vi "UDP Data Link - Driver Utilities - Asynch UDP Loop.vi"(11 "Input Data":T1) -> ()   [LabVIEW 2012, in "UDP Data Link Engine.lvlib"]
doc: "This VI is launched dynamically in its own memory space from the inline model VI. Before running, the Input Data control is initialized with UDP information entered by the user in System Explorer and with the appropriate RT FIFOs and Status Notifier.\n\nThis VI waits for data from an RT FIFO, converts the data to the appropriate packet data, and writes the packet over UDP to a Simulation Machine. The Simulation Machine responds with a UDP packet of its own, which this VI is monitoring in a separate loop. Upon receving UDP packets, this VI converts it to the appropriate data, determines any errors, and writes this data to the inline model VI via RT FIFO."
uses:
  UDP Data Link Engine.lvlib
  <vilib>/NI Veristand/Custom Device Tools/Custom Device Utility Library/Custom Device Utility Library.lvlib
panel:
  in  "Protocol Info":cluster{"ProtocolId":u8, "ProtocolRev":u8}={"ProtocolId"=1, "ProtocolRev"=16} {"ProtocolRev" format="%b"; "ProtocolId" format="%b"}
  # "If protocol info is rev'd, modify this cluster and then save as defualut data."
  # "From RT Driver VI"
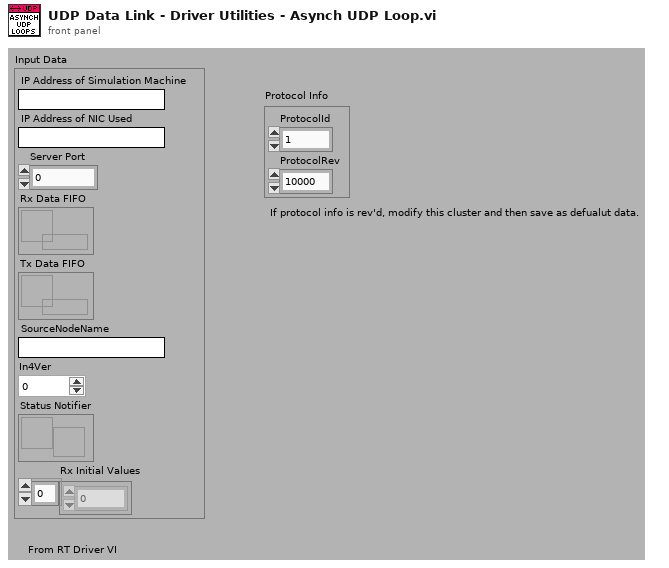
[diagram p1: front panel]
types:
  T1 = cluster{"IP Address of Simulation Machine":string, "IP Address of NIC Used":string, "Server Port":u16, "Rx Data FIFO":refnum<k33>, "Tx Data FIFO":refnum<k33>, "SourceNodeName":string, "In4Ver":u16, "Status Notifier":refnum<notifier>, "Rx Initial Values":dbl[]}
  T2 = enum16{"big-endian, network order", "native, host order", "little-endian"}
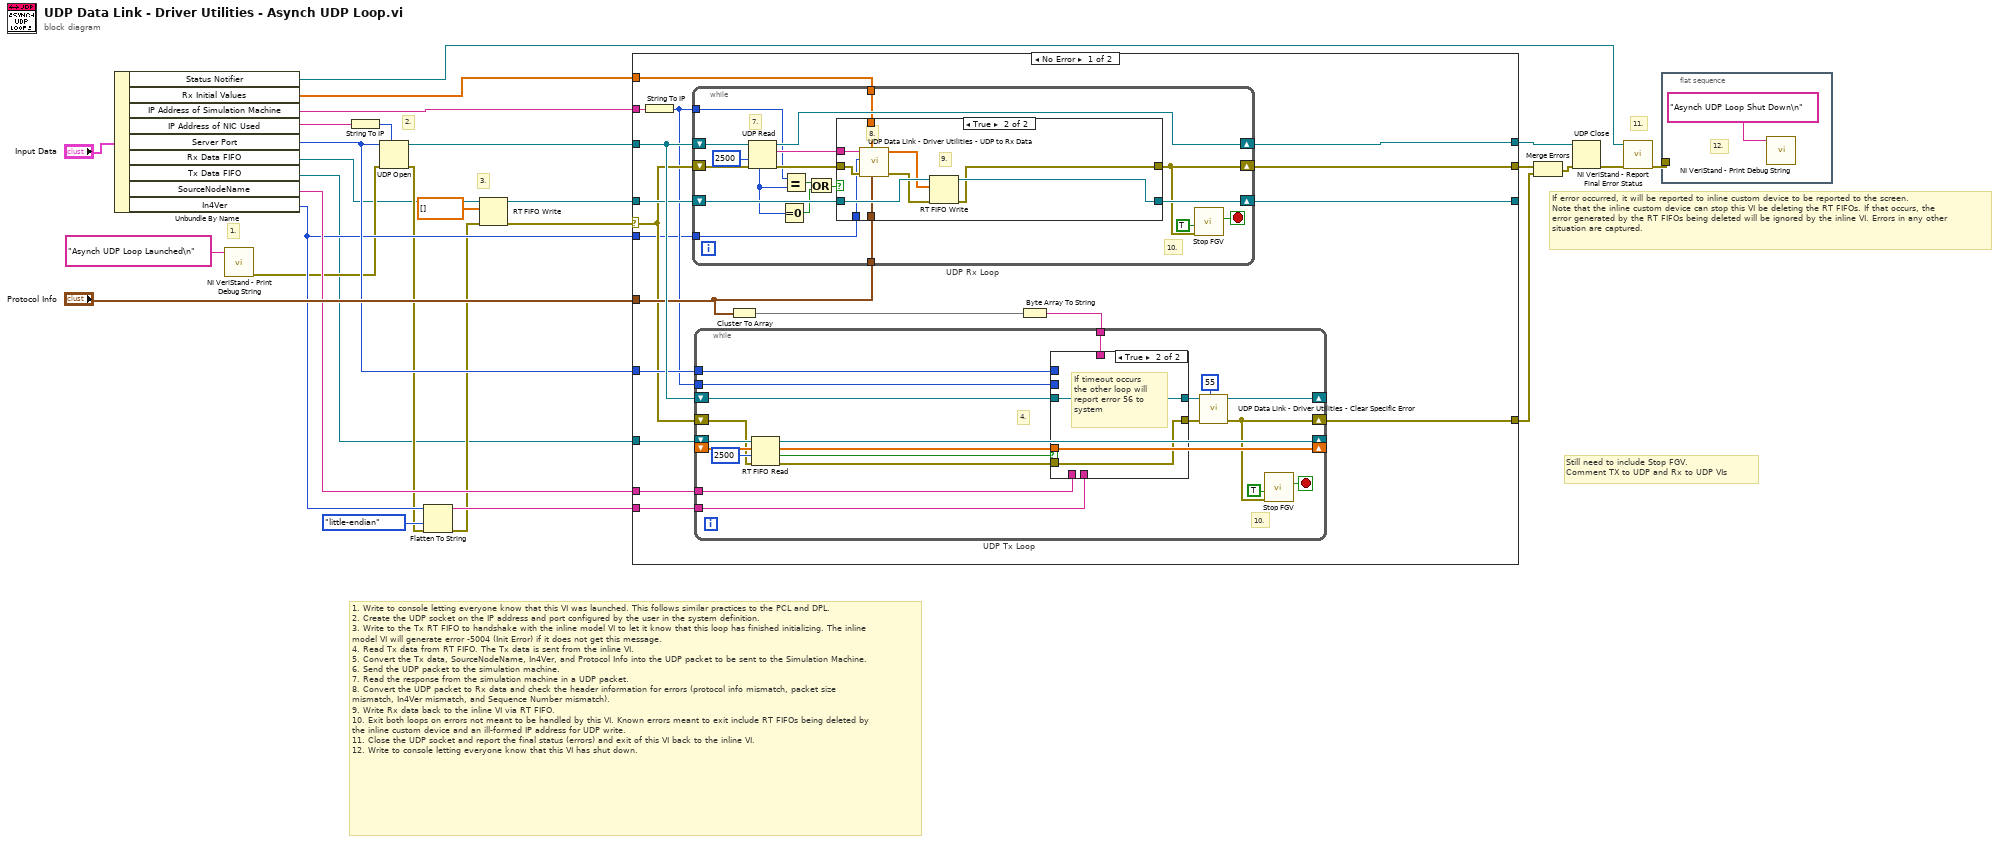
[diagram p0: block diagram]
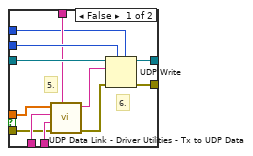
[diagram p2: hidden frame]
diagram:
  # "Still need to include Stop FGV.\nComment TX to UDP and Rx to UDP VIs"
  # "11."
  # "1. Write to console letting everyone know that this VI was launched. This follows similar practices to the PCL and DPL.\n2. Create the UDP socket on the IP address and port configured by the user in the system definition.\n3. Write to the Tx RT FIFO to handshake with the inline model VI to let it know that this loop has finished initializing. The inline model VI will generate error -5004 (Init Error) if it does not get this message.\n4. Read Tx data from RT FIFO. The Tx data is sent from the inline VI.\n5. Convert the Tx data, SourceNodeName, In4Ver, and Protocol Info into the UDP packet to be sent to the Simulation Machine.\n6. Send the UDP packet to the simulation machine.\n7. Read the response from the simulation machine in a UDP packet.\n8. Convert the UDP packet to Rx data and check the header information for errors (protocol info mismatch, packet size mismatch, In4Ver mismatch, and Sequence Number mismatch).\n9. Write Rx data back to the inline VI via RT FIFO.\n10. Exit both loops on errors not meant to be handled by this VI. Known errors meant to exit include RT FIFOs being deleted by the inline custom device and an ill-formed IP address for UDP write.\n11. Close the UDP socket and report the final status (errors) and exit of this VI back to the inline VI.\n12. Write to console letting everyone know that this VI has shut down."
  # "3."
  # "2."
  # "1."
  # "If error occurred, it will be reported to inline custom device to be reported to the screen.\nNote that the inline custom device can stop this VI be deleting the RT FIFOs. If that occurs, the error generated by the RT FIFOs being deleted will be ignored by the inline VI. Errors in any other situation are captured."
  n1 = Unbundle By Name("Input Data") -> ("Status Notifier"=w3:refnum<notifier>, "Rx Initial Values"=w2:dbl[], "IP Address of Simulation Machine"=w17:string, "IP Address of NIC Used"=w27:string, "Server Port"=w15:u16, "Rx Data FIFO"=w5:refnum<k33>, "Tx Data FIFO"=w4:refnum<k33>, "SourceNodeName"=w24:string, "In4Ver"=w14:u16)
  n2 = call <vilib>:"NI VeriStand - Print Debug String.vi"("Message"="Asynch UDP Loop Launched\n" ("String to write")) -> ("error out"=w8:errorcluster)  [unwired: 10 in]
  n3 = String To IP(1:w27) -> (0:w16:u32)
  n4 = UDP Open(7:w16, 8:w8, 11:w15) -> (port=w26:refnum<k16>, 0:w7:errorcluster)  [unwired: 2 in, 1 out]
  n5 = Flatten To String(anything=w14, byte order (0:big-endian, network order)=T2."little-endian", error in (no error)=w7) -> (data string=w23:string, error out=w6:errorcluster)  [unwired: 1 in, 1 out]
  n6 = RT FIFO Write(0:w5, 1:dbl[] [] ("element"), 3:w6) -> (8:w21:refnum<k33>, 11:w1:errorcluster)  [unwired: 2 in, 2 out]
  n7 = case shown="No Error" w1 {
    selector: w1 -> [w37 w113]
    tunnel: w26 -> [w46 w114]
    tunnel: w4 -> [w45 _]
    tunnel: w17 -> [w35 _]
    tunnel: "Protocol Info" -> [w44 _]
    tunnel: w24 -> [w41 _]
    tunnel: w23 -> [w40 _]
    tunnel: w15 -> [w39 _]
    tunnel: w21 -> [w38 w112]
    tunnel: [w36 w114] -> w18
    tunnel: w14 -> [w33 _]
    tunnel: [w32 w113] -> w13
    tunnel: [w31 w113] -> w12
    tunnel: [w30 w112] -> _
    tunnel: w2 -> [w29 _]
    frame No Error {
      n8 = String To IP(1:w35) -> (0:w34:u32)
      n9 = while "UDP Rx Loop" {
        shift-right: [w83] -> w32
        shift-left: w37 -> [w91]
        shift-right: [w93] -> w30
        shift-left: w38 -> [w98]
        shift-right: [w94] -> w36
        shift-left: w46 -> [w99]
        tunnel: w34 -> [w90]
        tunnel: w44 -> [w92]
        tunnel: w33 -> [w89]
        tunnel: w29 -> [w84]
        stop <- w82 stop-if-true
        # "10."
        # "7."
        n10 = UDP Read(connection ID=w99, timeout ms (25000)=2500, 8:w91) -> (data out=w95:string, error out=w96:errorcluster, 3:w94:refnum<k16>, 6:w85:u32)  [unwired: 1 in, 1 out]
        n11 = Equal To 0?(x=w85) -> (x = 0?=w86:bool)
        n12 = Equal?(x=w90, y=w85) -> (x = y?=w87:bool)
        n13 = Or(x=w87, y=w86) -> (x .or. y?=w88:bool)
        n14 = case shown="True" w88 {
          tunnel: w98 -> [w101 w111]
          tunnel: w96 -> [w100 w108]
          tunnel: w95 -> [_ w109]
          tunnel: [w101 w110] -> w93
          tunnel: [w100 w102] -> w83
          tunnel: w92 -> [_ w105]
          tunnel: w89 -> [_ w104]
          tunnel: w84 -> [_ w103]
          frame False {
          }
          frame True {
            # "9."
            # "8."
            n15 = call "UDP Data Link - Driver Utilities - UDP to Rx Data.vi"("Protocol Info"=w105, "Rx Initial Values"=w103, "error in (no error)"=w108, "In4Ver"=w104, "UDP Data"=w109) -> ("error out"=w106:errorcluster, "Rx Data"=w107:dbl[])  [unwired: 4 in, 1 out]
            n16 = RT FIFO Write(0:w111, 1:w107, 3:w106) -> (8:w110:refnum<k33>, 11:w102:errorcluster)  [unwired: 2 in, 2 out]
          }
        }
        n17 = call "Stop FGV.vi"("error in (no error)"=w83, "Stop on Error?"=TRUE) -> ("Latched Stop"=w82:bool)  [unwired: 7 in, 2 out]
      }
      n18 = Cluster To Array(cluster=w44) -> (array=w43:u8[])
      n19 = Byte Array To String(unsigned byte array=w43) -> (string=w42:string)
      n20 = while "UDP Tx Loop" {
        shift-right: [w48] -> w31
        shift-left: w37 -> [w53]
        shift-right: [w61] -> _
        shift-left: w45 -> [w66]
        shift-right: [w55] -> _
        shift-left: w46 -> [w64]
        tunnel: w34 -> [w65]
        shift-right: [w59] -> _
        shift-left: _ -> [w62]
        tunnel: w42 -> [w58]
        tunnel: w41 -> [w57]
        tunnel: w40 -> [w56]
        tunnel: w39 -> [w54]
        stop <- w51 stop-if-true
        # "10."
        # "4."
        n21 = RT FIFO Read(0:w66, 1:w62, 2:2500 ("timeout in ms (0)"), 3:w53) -> (8:w61:refnum<k33>, 9:w59:dbl[], 10:w60:bool, 11:w47:errorcluster)  [unwired: 1 out]
        n22 = case shown="True" w60 {
          tunnel: w65 -> [w78 _]
          tunnel: w64 -> [w77 w80]
          tunnel: w59 -> [w75 _]
          tunnel: [w76 w79] -> w49
          tunnel: w58 -> [w72 _]
          tunnel: w57 -> [w71 _]
          tunnel: w56 -> [w70 _]
          tunnel: [w69 w80] -> w55
          tunnel: w54 -> [w68 _]
          tunnel: w47 -> [w67 w79]
          frame False {
            # "6."
            # "5."
            n23 = call "UDP Data Link - Driver Utilities - Tx to UDP Data.vi"("Protocol Info"=w72, "error in (no error)"=w67, "In4Ver"=w70, "SourceNodeName"=w71, "Tx Data"=w75) -> ("error out"=w73:errorcluster, "UDP Data"=w74:string)  [unwired: 5 in]
            n24 = UDP Write(address=w78, port or service name=w68, connection ID=w77, data in=w74, 8:w73) -> (error out=w76:errorcluster, 3:w69:refnum<k16>)  [unwired: 1 in]
          }
          frame True {
            # "If timeout occurs the other loop will report error 56 to system"
          }
        }
        n25 = call "UDP Data Link - Driver Utilities - Clear Specific Error.vi"("Error to Clear"=55, "Error In"=w49) -> ("Error Out"=w48:errorcluster)  [unwired: 6 in, 1 out]
        n26 = call "Stop FGV.vi"("error in (no error)"=w48, "Stop on Error?"=TRUE) -> ("Latched Stop"=w51:bool)  [unwired: 7 in, 2 out]
      }
    }
    frame Error {
    }
  }
  n27 = Merge Errors(w13, w12) -> (w11:errorcluster)
  n28 = UDP Close(connection ID=w18, 8:w11) -> (error out=w10:errorcluster)  [unwired: 1 out]
  n29 = call <vilib>:"NI VeriStand - Report Final Error Status.vi"("error in (no error)"=w10, "Status Notifier"=w3) -> ("error out"=w9:errorcluster)  [unwired: 9 in]
  n30 = flat-sequence {
    tunnel: w9 -> [_]
    frame #0 {
      # "12."
      n31 = call <vilib>:"NI VeriStand - Print Debug String.vi"("Message"="Asynch UDP Loop Shut Down\n" ("String to write")) -> ()  [unwired: 10 in, 1 out]
    }
  }
